vi "GFG_Monitor.vi"(8 "error in (no error)":errorcluster) -> (0 "error out":errorcluster)   [LabVIEW 2012, in "GFG library.lvlib"]
doc: "SciScan 1.2 160622\nThis VI implements a diagnostic tool to probe the value of a GFG variable and gives details such as modifying VI, latest value, etc"
uses:
  GFG library.lvlib
panel:
  out "Variant value (on last refresh)":variant
  in  "clear":bool
  in  "Index":dbl
  out "Variables (array of clusters)":cluster{u32[], string[], string[], variant[]}
  in  "Query Variable":string
  in  "Refresh":bool
  out "All Variables":string[](array[string])
  in  "stop":bool
  # "Time since previous\nvariable change (in ms)"
  # "Variable Name"
  # "Caller"
  # "Variant Value"
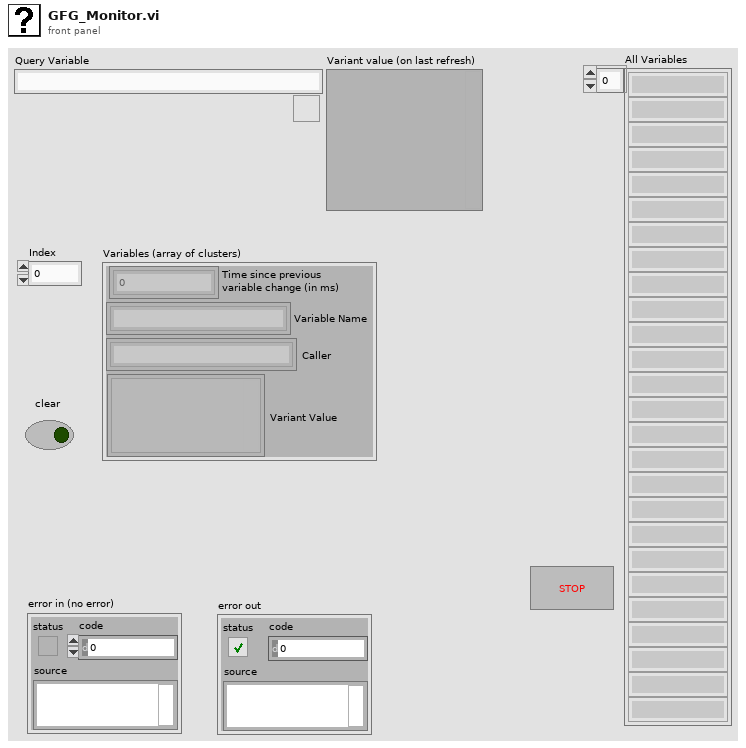
[diagram p1: front panel]
types:
  T1 = typedef "VariantType.lvlib/Type.ctl" = enum8{"Invalid Type", "Void", "I8", "I16", "I32", "I64", "U8", "U16", "U32", "U64", "Single Float", "Double Float", "Extended Float", "Single Complex", "Double Complex", "Extended Complex", "Enum U8", "Enum U16", "Enum U32", "Enum U64", "Single Float With Unit", "Double Float With Unit", "Extended Float With Unit", "Single Complex with Unit", "Double Complex with Unit", "Extended Complex with Unit", "Boolean", "String", "Path", "Picture", "Tag", "Array", "Cluster", "Variant", "LV Variant", "Waveform", "Timestamp", "Digital Waveform", "Digital Data", "ExpressData", "Refnum", "External Data", "VI", "Poly VI", "LabVIEW Class Instance", "Fixed Point"}
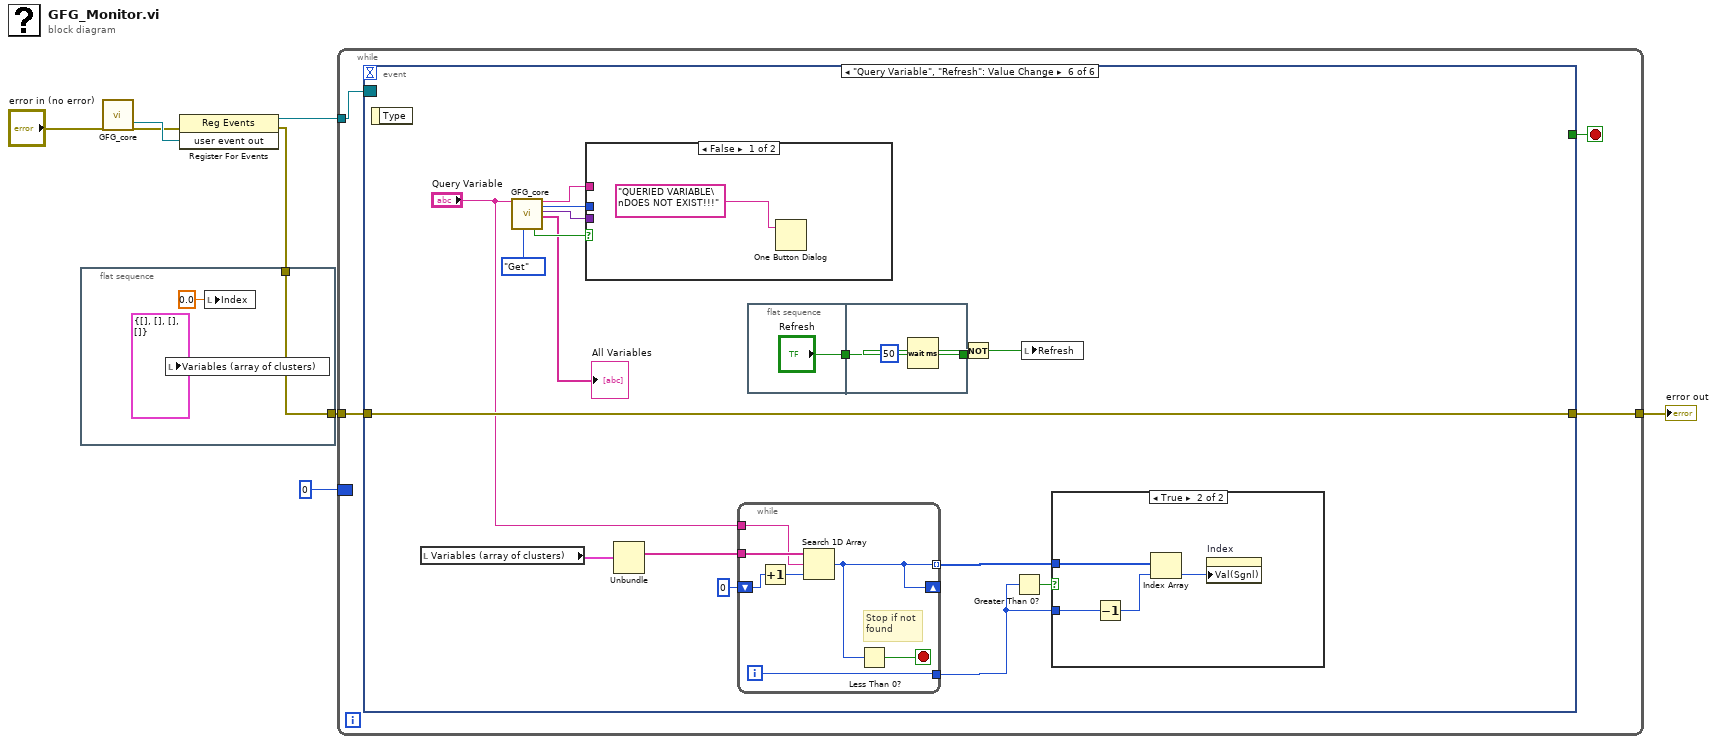
[diagram p0: block diagram]
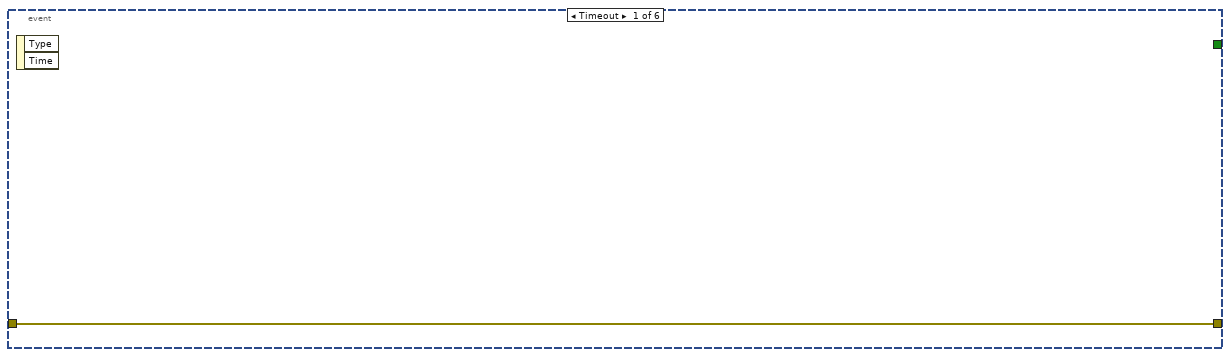
[diagram p2: hidden frame]
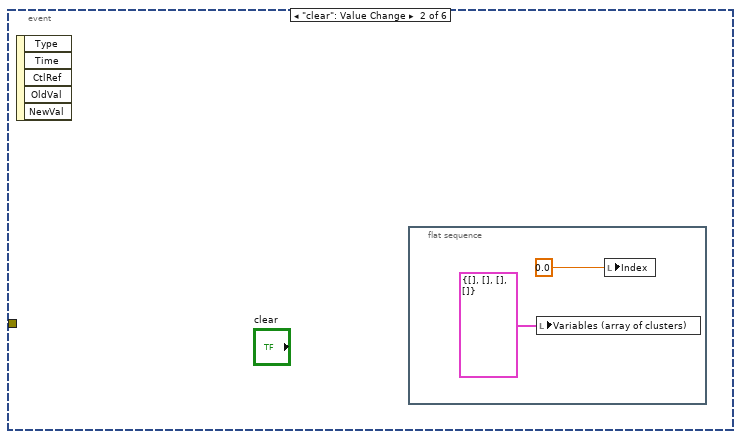
[diagram p3: hidden frame]
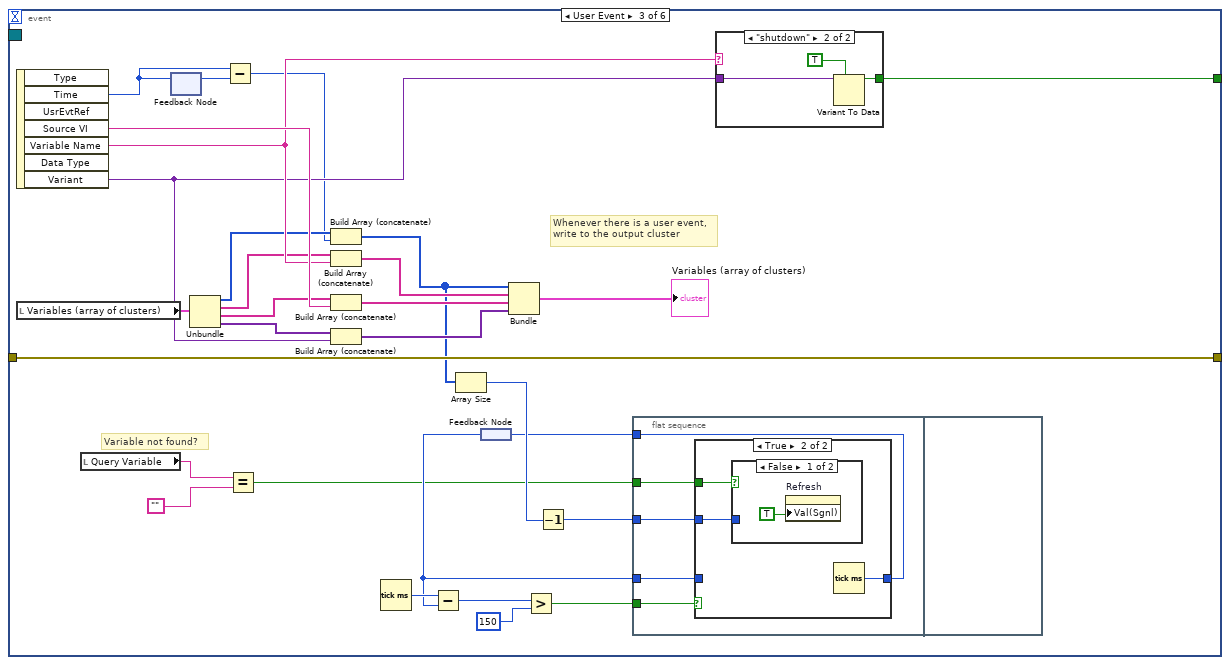
[diagram p4: hidden frame]
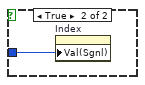
[diagram p6: hidden frame]
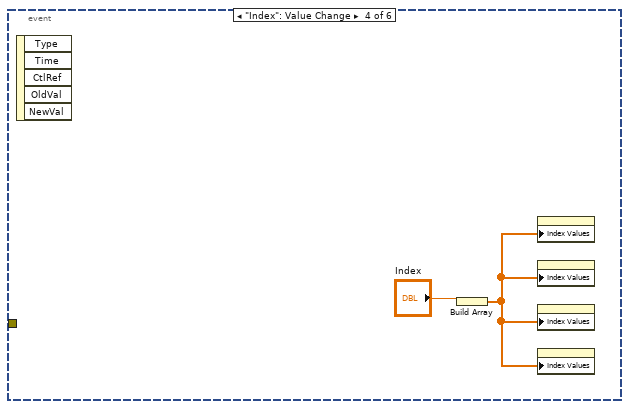
[diagram p8: hidden frame]
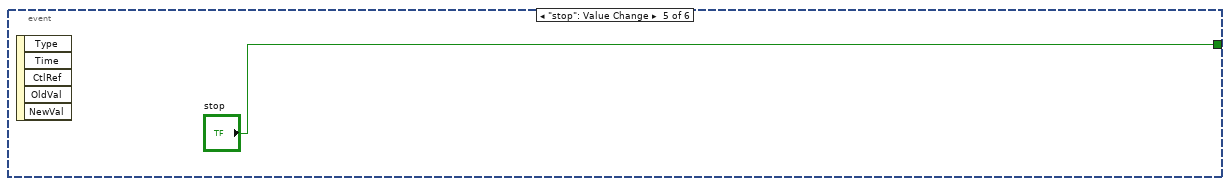
[diagram p9: hidden frame]
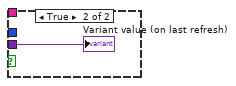
[diagram p11: hidden frame]
diagram:
  n1 = flat-sequence {
    tunnel: [w10] -> w3
    tunnel: w2 -> [w10]
    frame #0 {
      n2 = local write "Variables (array of clusters)"(cluster{u32[], string[], string[], variant[]} {[], [], [], []} ("output cluster")) -> ()
      n3 = local write "Index"(0.0 ("Index")) -> ()
    }
  }
  n4 = call "GFG_core.vi"("error in (no error)"="error in (no error)") -> ("user event out"=w7:refnum<user-event>, "error out"=w6:errorcluster)  [unwired: 12 in, 5 out]
  n5 = register-events(error in=w6, w7) -> (reference out=w8:refnum<event-registration>, error out=w2:errorcluster)  [unwired: 1 in]
  n6 = while {
    tunnel: w8 -> [w15]
    tunnel: w3 -> [w13]
    tunnel: [w12] -> w4
    border: u32 0 ("millisecond timer value") -> [_]
    stop <- w14 stop-if-true
    n7 = event shown="[5] \"Query Variable\", \"Refresh\": Value Change" {
      selector: w15 -> [_ _ _ _ _ _]
      dyn-events: _ -> [_ _ _ _ _ _]
      timeout: _ -> [_ _ _ _ _ _]
      tunnel: [_ _ w47 _ "stop" _] -> w14
      tunnel: w13 -> [w16 _ w46 _ _ w75]
      tunnel: [w16 _ w46 _ _ w75] -> w12
      event Timeout {
        n8 = event-data() -> ()  [unwired: 1 in, 2 out]
      }
      event "clear": Value Change {
        n9 = event-data() -> ()  [unwired: 1 in, 5 out]
        n10 = flat-sequence {
          frame #0 {
            n11 = local write "Variables (array of clusters)"(cluster{u32[], string[], string[], variant[]} {[], [], [], []} ("output cluster")) -> ()
            n12 = local write "Index"(0.0 ("Index")) -> ()
          }
        }
      }
      event User Event {
        # "Whenever there is a user event,\nwrite to the output cluster"
        # "Variable not found?"
        n13 = event-data() -> ("Time"=w21:u32, "Source VI"=w45:string, "Variable Name"=w44:string, "Variant"=w43:variant)  [unwired: 1 in, 3 out]
        n14 = local read "Variables (array of clusters)"() -> (w38:cluster{u32[], string[], string[], variant[]})
        n15 = local read "Query Variable"() -> (w24:string)
        n16 = feedback-in #1(w21) -> ()
        n17 = feedback #1() -> (w20:u32)  [unwired: 1 in]
        n18 = Unbundle(w38) -> (w37:u32[], w36:string[], w35:string[], w34:variant[])
        n19 = Subtract(x=w21, y=w20) -> (x-y=w19:u32)
        n20 = Equal?(x=w24, y="") -> (x = y?=w22:bool)
        n21 = Build Array (concatenate)(w37, w19) -> (w33:u32[])
        n22 = Build Array (concatenate)(w36, w44) -> (w42:string[])
        n23 = Build Array (concatenate)(w35, w45) -> (w40:string[])
        n24 = Build Array (concatenate)(w34, w43) -> (w41:variant[])
        n25 = Tick Count (ms)() -> (millisecond timer value=w29:u32)
        n26 = Array Size(array=w33) -> (size(s)=w32:i32)
        n27 = feedback-in #2(w30) -> ()
        n28 = feedback #2() -> (w25:u32)
        n29 = Subtract(x=w29, y=w25) -> (x-y=w28:u32)
        n30 = Bundle(w33, w42, w40, w41) -> (→"Variables (array of clusters)":cluster{u32[], string[], string[], variant[]})  [unwired: 1 in]
        n31 = Greater?(x=w28, y=u32 150) -> (0:w26:bool)
        n32 = Decrement(x=w32) -> (x-1=w31:i32)
        n33 = flat-sequence {
          tunnel: w31 -> [w52]
          tunnel: [w51] -> w30
          tunnel: w26 -> [w50]
          tunnel: w25 -> [w49]
          tunnel: w22 -> [w48]
          frame #0 {
            n34 = case shown="True" w50 {
              tunnel: w52 -> [_ w56]
              tunnel: [w53 w55] -> w51
              tunnel: w49 -> [w53 _]
              tunnel: w48 -> [_ w54]
              frame False {
              }
              frame True {
                n35 = case shown="False" w54 {
                  tunnel: w56 -> [_ w58]
                  frame False {
                    n36 = property on="Refresh" class="Bool (strict)"("Val(Sgnl)"=TRUE ("Refresh")) -> ()  [unwired: 2 in, 2 out]
                  }
                  frame True {
                    n37 = property on="Index" class="DigNum (strict)"("Val(Sgnl)"=w58) -> ()  [unwired: 2 in, 2 out]
                  }
                }
                n38 = Tick Count (ms)() -> (millisecond timer value=w55:u32)
              }
            }
          }
          frame #1 {
          }
        }
        n39 = case shown="\"shutdown\"" w44 {
          tunnel: w43 -> [_ w61]
          tunnel: [_ w59] -> w47
          frame "False", Default {
          }
          frame "shutdown" {
            n40 = Variant To Data(type=TRUE ("want seconds? (F)"), Variant=w61) -> (data=w59:bool)  [unwired: 1 in, 1 out]
          }
        }
      }
      event "Index": Value Change {
        n41 = event-data() -> ()  [unwired: 1 in, 5 out]
        n42 = Build Array("Index") -> (w62:dbl[])
        n43 = property class="Arr (strict)"("Index Values"=w62) -> ()  [unwired: 2 in, 2 out]
        n44 = property class="Arr (strict)"("Index Values"=w62) -> ()  [unwired: 2 in, 2 out]
        n45 = property class="Arr (strict)"("Index Values"=w62) -> ()  [unwired: 2 in, 2 out]
        n46 = property class="Arr (strict)"("Index Values"=w62) -> ()  [unwired: 2 in, 2 out]
      }
      event "stop": Value Change {
        n47 = event-data() -> ()  [unwired: 1 in, 5 out]
      }
      event "Query Variable", "Refresh": Value Change {
        n48 = event-data() -> ()  [unwired: 1 in, 1 out]
        n49 = local read "Variables (array of clusters)"() -> (w74:cluster{u32[], string[], string[], variant[]})
        n50 = call "GFG_core.vi"("Variable Name in"="Query Variable", "Action"=enum16{"Init", "Set", "Get"}."Get") -> ("Found/Replaced"=w77:bool, "Variable Name Out"=w80:string, "Data Type Out"=w78:T1, "Variant Out"=w79:variant, "All Variable Names Out"=→"All Variables":string[])  [unwired: 11 in, 2 out]
        n51 = case shown="False" w77 {
          tunnel: w80 -> [_ _]
          tunnel: w79 -> [_ w97]
          tunnel: w78 -> [_ _]
          frame False {
            n52 = One Button Dialog(message="QUERIED VARIABLE\nDOES NOT EXIST!!!" ("Variable Name Out")) -> ()  [unwired: 1 in, 1 out]
          }
          frame True {
            "Variant value (on last refresh)" <- w97
          }
        }
        n53 = Unbundle(w74) -> (w73:string[])  [unwired: 3 out]
        n54 = while {
          tunnel: w73 -> [w95]
          tunnel: "Query Variable" -> [w94]
          tunnel: [w91] -> w71 mode=indexing
          tunnel: [w92] -> w69
          shift-right: [w91] -> _
          shift-left: 0 ("index of element") -> [w90]
          i -> [w92]
          stop <- w93 stop-if-true
          # "Stop if not\nfound"
          n55 = Increment(x=w90) -> (x+1=w89:i32)
          n56 = Search 1D Array(1D array=w95, element=w94, start index (0)=w89) -> (index of element=w91:i32)
          n57 = Less Than 0?(x=w91) -> (x < 0?=w93:bool)
        }
        n58 = flat-sequence {
          tunnel: ["Refresh"] -> w65
          tunnel: [w84] -> w67
          tunnel: w65 -> [w84]
          frame #0 {
          }
          frame #1 {
            n59 = Wait (ms)(milliseconds to wait=u32 50) -> ()  [unwired: 1 out]
          }
        }
        n60 = Not(x=w67) -> (.not. x?=w66:bool)
        n61 = Greater Than 0?(x=w69) -> (x > 0?=w70:bool)
        n62 = local write "Refresh"(w66) -> ()
        n63 = case shown="True" w70 {
          tunnel: w71 -> [_ w88]
          tunnel: w69 -> [_ w87]
          frame False {
            # "The queried element not found!"
          }
          frame True {
            n64 = Decrement(x=w87) -> (x-1=w86:i32)
            n65 = Index Array(array=w88, index=w86) -> (element=w85:i32)
            n66 = property on="Index" class="DigNum (strict)"("Val(Sgnl)"=w85) -> ()  [unwired: 2 in, 2 out]
          }
        }
      }
    }
  }
  "error out" <- w4
